vi "IIR Cascade Filter (CDB).vi"(2 "init/cont (init:F)":bool, 3 "IIR Filter Cluster":T1 {"Forward Coefficients" format="%.4f"; "Reverse Coefficients" format="%.4f"}, 4 "X":cdb[](array[numeric])) -> (0 "error":i32, 1 "Filtered X":cdb[](array[numeric]))   [LabVIEW 2014, in "NI_AALBase.lvlib"]
doc: "Filters the input sequence <B>X</B> using the cascade form of the IIR filter specified by the <B>IIR Filter Cluster</B>. Wire data to the <B>X</B> input to determine the polymorphic instance to use or manually select the instance."
uses:
  NI_AALBase.lvlib
  lvanlys.dll
panel:
  in  "shift register type":cdb[](array[numeric]) format="%0.2f"
  # "IIR Cascade\nFilter"
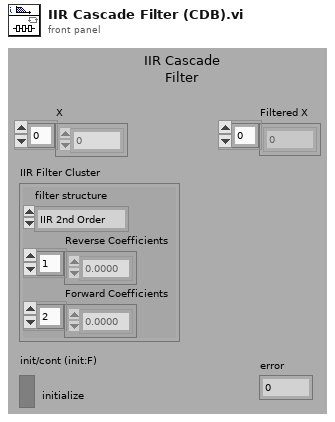
[diagram p1: front panel]
types:
  T1 = cluster{"filter structure":enum32{"IIR 2nd Order", "IIR 4th Order"}, "Reverse Coefficients":dbl[], "Forward Coefficients":dbl[]}
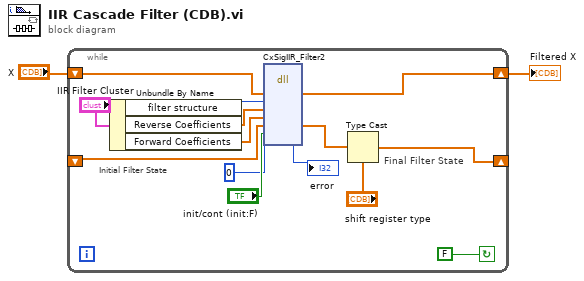
[diagram p0: block diagram]
diagram:
  n1 = while {
    shift-left: _ -> [w11]
    shift-right: [w16] -> _
    shift-right: [w3] -> w1
    shift-left: "X" -> [w4]
    stop <- FALSE continue-if-true
    # "Final Filter State"
    # "Initial Filter State"
    n2 = Unbundle By Name("IIR Filter Cluster") -> ("filter structure"=w14:enum32{"IIR 2nd Order", "IIR 4th Order"}, "Reverse Coefficients"=w13:dbl[], "Forward Coefficients"=w12:dbl[])
    n3 = dll-call lib="C:/Program Files (x86)/National Instruments/LabVIEW 2014/resource/lvanlys.*" fn="CxSigIIR_Filter2"("X"=w4, "filter structure"=w14, "aH"=w13, "bH"=w12, "shift register type"=w11, "init/cont (init:F)"="init/cont (init:F)", 0) -> ("X"=w3:cdb[], "shift register type"=w9:cdb[], →"error":i32)  [unwired: 8 in, 2 out]
    n4 = Type Cast(type="shift register type", x=w9) -> (*(type *) &x=w16:cdb[])
  }
  "Filtered X" <- w1
